vi "Simple example.vi"() -> ()   [LabVIEW 2020]
uses:
  shared/OnOffTypeDef.ctl
  Serial Commands Slink.ctl
  Gentec SlinkUSB.lvclass
panel:
  out "Measure":dbl format="%.3e"
  out "String":string
  in  "stop new":bool
  out "Ch 2 out":dbl format="%.6f"
  in  "error in (no error)":errorcluster
  out "Channel 1 value":dbl
  out "Channel 2 value":dbl
  out "Message Based Settings:Termination Character":u8=10 format="%x"
  out "read buffer 5":string
  out "read buffer 4":string
  out "read buffer 3":string
  out "read buffer 2":string
  out "return count 3":u32
  out "return count 2":u32
  out "Scale Ch":dbl format="%^.0e"
  out "Ext Trig":string
  out "Wavelength":string="0"
  out "error out":errorcluster={"status"=TRUE, "code"=-1073807339, "source"="VISA Read in slink read energy w termination chars.vi->Simple example.vi"}
  out "read buffer":string
  in  "stop":bool
  in  "time to reset":i32=1000
  in  "ChannelEnable":cluster{"Channel 1":T1, "Channel 2":T1}={"Channel 1"=enum."on", "Channel 2"=enum."on"}
  in  "devport":string="COM5"
  out "VISA Refnum out":refnum<visa-resource-name>="COM5"
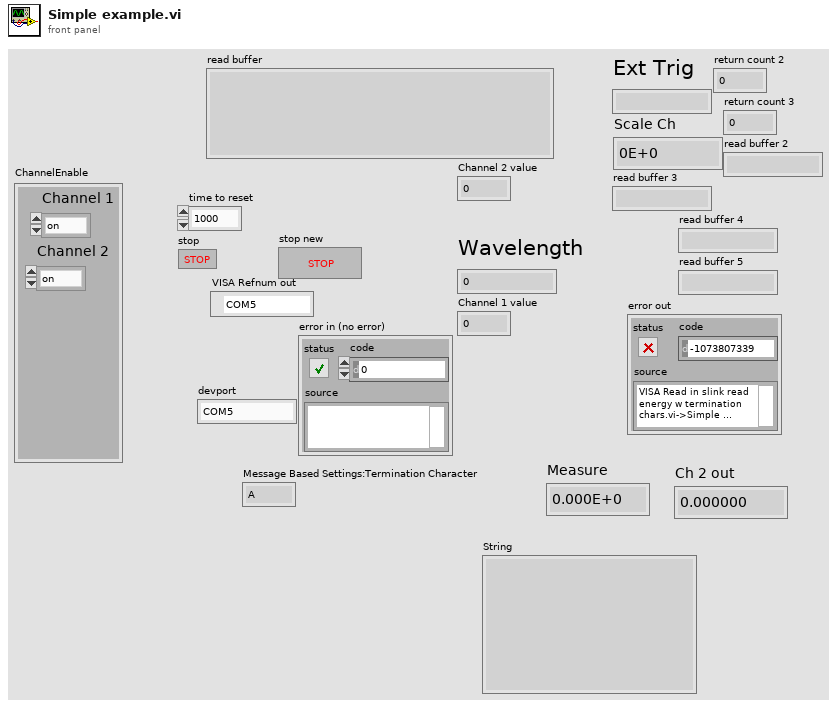
[diagram p1: front panel]
types:
  T1 = typedef "OnOffTypeDef.ctl" = enum16{"off", "on"}
  T2 = typedef "Serial Commands Slink.ctl" = i32
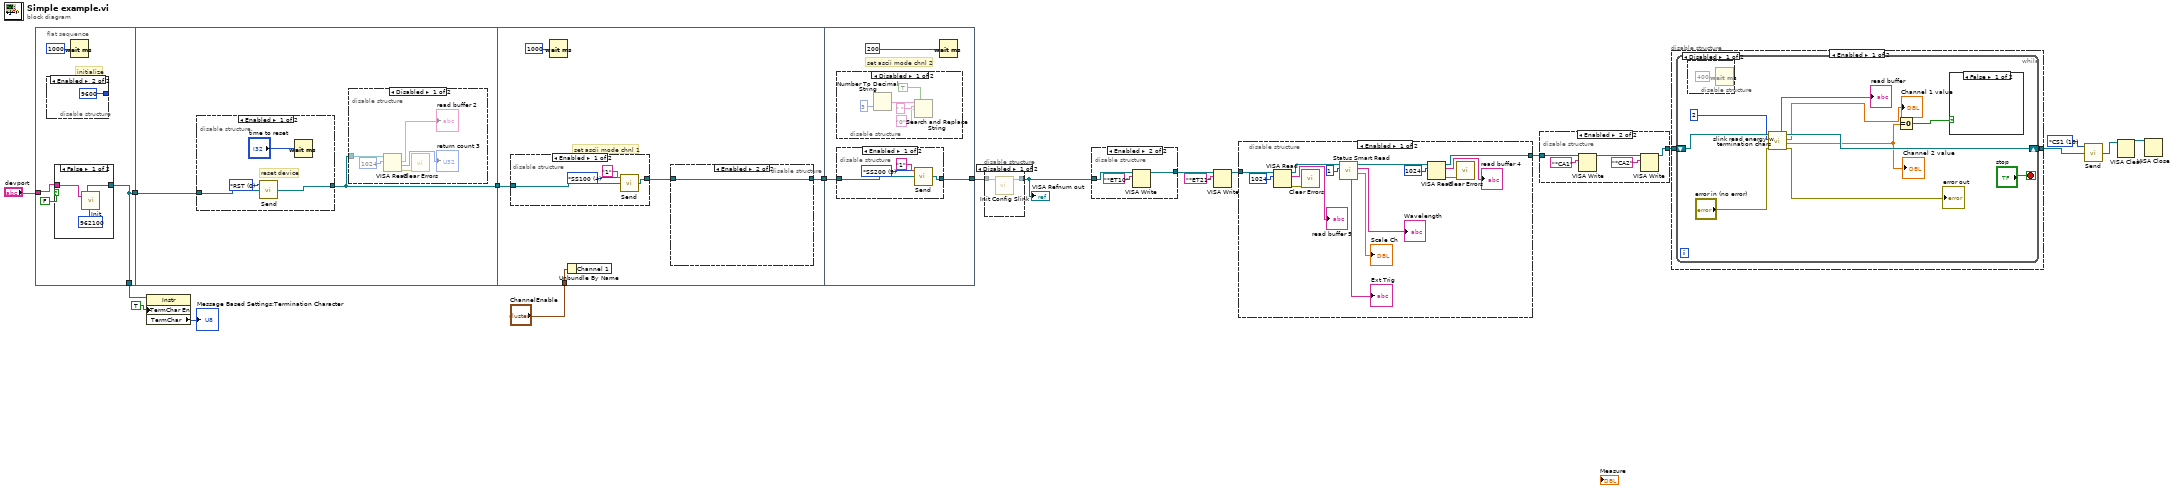
[diagram p0: block diagram]
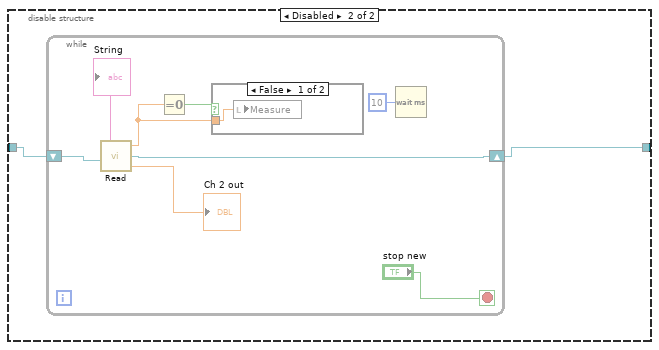
[diagram p4: hidden frame]
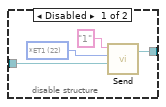
[diagram p7: hidden frame]
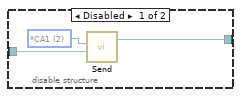
[diagram p9: hidden frame]
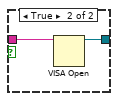
[diagram p10: hidden frame]
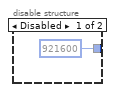
[diagram p11: hidden frame]
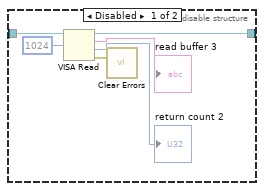
[diagram p14: hidden frame]
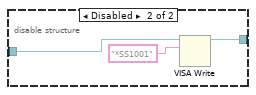
[diagram p15: hidden frame]
diagram:
  w11 = 10 items=["*RST", "*VER", "*CA1", "*CA2", "*SS1", "*SS2", "*SU1", "*SU2", "*SD1", "*SD2", "*CS1", "*CS2", "*AT1", "*AT2", "*AN1", "*AN2", "*PW1", "*PW2", "*TL1", "*TL2", "*ST1", "*ST2", "*ET1", "*ET2", "*EM1", "*EM2", "*SC1", "*SC2"] ("string to write")
  n1 = flat-sequence {
    tunnel: "devport" -> [w22]
    tunnel: [w21] -> w19
    tunnel: [w21] -> w6
    tunnel: w19 -> [w32]
    tunnel: [w31] -> w18
    tunnel: w18 -> [w46]
    tunnel: [w43] -> w17
    tunnel: "ChannelEnable" -> [w45]
    tunnel: [w63] -> w14
    tunnel: w17 -> [w62]
    frame #0 {
      # "initialize"
      n2 = disable-structure shown="Enabled" {
        disable-tunnel: [u32 921600 ("Baud Rate 3") u32 9600 ("Baud Rate 2")] -> _
        frame Disabled {
        }
        frame Enabled {
        }
      }
      n3 = case shown="False" FALSE {
        tunnel: w22 -> [w26 w28]
        tunnel: [w25 w27] -> w21
        frame False {
          n4 = call "Init.vi"("Baud Rate 2"=u32 962100, "# Port"=w26) -> ("VISA resource name out"=w25:refnum<visa-resource-name>)
        }
        frame True {
          n5 = VISA Open(VISA resource name=w28) -> (VISA resource name=w27:refnum<visa-resource-name>)  [unwired: 4 in, 1 out]
        }
      }
      n6 = Wait (ms)(milliseconds to wait=1000) -> ()  [unwired: 1 out]
    }
    frame #1 {
      n7 = disable-structure shown="Enabled" {
        disable-tunnel: [w40 w42] -> w31
        disable-tunnel: w32 -> [w39 w42]
        frame Enabled {
          w38 = T2 0 items=["*RST", "*VER", "*CA1", "*CA2", "*SS100", "*SS200", "*SU1", "*SU2", "*SD1", "*SD2", "*CS1", "*CS2", "*AT1", "*AT2", "*AN1", "*AN2", "*PW1", "*PW2", "*TL1", "*TL2", "*ST1", "*ST2", "*ET1", "*ET2", "*EM1", "*EM2", "*SC1", "*SC2", "*VNM", "*CV1", "*CV2"] ("string to write")
          # "reset device"
          n8 = call "Send.vi"("string to write"=w38, "port number"=w39) -> ("VISA resource name out"=w40:refnum<visa-resource-name>)  [unwired: 2 in, 1 out]
          n9 = Wait (ms)(milliseconds to wait="time to reset") -> ()  [unwired: 1 out]
        }
        frame Disabled {
        }
      }
      n10 = disable-structure shown="Disabled" {
        disable-tunnel: w31 -> [w36 _]
        frame Disabled {
          n11 = VISA Read(VISA resource name=w36, byte count=u32 1024) -> (read buffer=→"read buffer 2":string, return count=→"return count 3":u32, error out=w35:errorcluster)  [unwired: 1 in, 1 out]
          n12 = call <vilib>:"Clear Errors.vi"("error in (no error)"=w35) -> ()  [unwired: 5 in, 2 out]
        }
        frame Enabled {
        }
      }
    }
    frame #2 {
      # "set ascii mode chnl 1"
      n13 = disable-structure shown="Enabled" {
        disable-tunnel: w46 -> [w58 w60]
        disable-tunnel: [w56 w59] -> w44
        frame Enabled {
          w55 = T2 4 items=["*RST", "*VER", "*CA1", "*CA2", "*SS100", "*SS200", "*SU1", "*SU2", "*SD1", "*SD2", "*CS1", "*CS2", "*AT1", "*AT2", "*AN1", "*AN2", "*PW1", "*PW2", "*TL1", "*TL2", "*ST1", "*ST2", "*ET1", "*ET2", "*EM1", "*EM2", "*SC1", "*SC2", "*VNM", "*CV1", "*CV2"] ("string to write")
          n14 = call "Send.vi"("string to write"=w55, "port number"=w58, "Option"="1") -> ("VISA resource name out"=w56:refnum<visa-resource-name>)  [unwired: 1 in, 1 out]
        }
        frame Disabled {
          n15 = VISA Write(VISA resource name=w60, write buffer="*SS1001") -> (VISA resource name out=w59:refnum<visa-resource-name>)  [unwired: 1 in, 2 out]
        }
      }
      n16 = Wait (ms)(milliseconds to wait=1000) -> ()  [unwired: 1 out]
      n17 = Unbundle By Name(w45) -> ()  [unwired: 1 out]
      n18 = disable-structure shown="Enabled" {
        disable-tunnel: w44 -> [w51 w54]
        disable-tunnel: [w48 w54] -> w43
        frame Disabled {
          n19 = VISA Read(VISA resource name=w51, byte count=u32 1024) -> (VISA resource name out=w48:refnum<visa-resource-name>, read buffer=→"read buffer 3":string, return count=→"return count 2":u32, error out=w52:errorcluster)  [unwired: 1 in]
          n20 = call <vilib>:"Clear Errors.vi"("error in (no error)"=w52) -> ()  [unwired: 5 in, 2 out]
        }
        frame Enabled {
        }
      }
    }
    frame #3 {
      # "set ascii mode chnl 2"
      n21 = disable-structure shown="Disabled" {
        frame Disabled {
          n22 = Number To Decimal String(width (-)=i16 3) -> (decimal integer string=w73:string)  [unwired: 1 in]
          n23 = Search and Replace String(replace all?=TRUE ("replace all? (F)"), input string=w73, search string=" ", replace string="0" ("replace string (\"\")")) -> ()  [unwired: 4 in, 4 out]
        }
        frame Enabled {
        }
      }
      n24 = disable-structure shown="Enabled" {
        disable-tunnel: [w68 w69] -> w63
        disable-tunnel: w62 -> [w67 w69]
        frame Enabled {
          w65 = T2 5 items=["*RST", "*VER", "*CA1", "*CA2", "*SS100", "*SS200", "*SU1", "*SU2", "*SD1", "*SD2", "*CS1", "*CS2", "*AT1", "*AT2", "*AN1", "*AN2", "*PW1", "*PW2", "*TL1", "*TL2", "*ST1", "*ST2", "*ET1", "*ET2", "*EM1", "*EM2", "*SC1", "*SC2", "*VNM", "*CV1", "*CV2"] ("string to write")
          n25 = call "Send.vi"("string to write"=w65, "port number"=w67, "Option"="1" ("search string")) -> ("VISA resource name out"=w68:refnum<visa-resource-name>)  [unwired: 1 in, 1 out]
        }
        frame Disabled {
        }
      }
      n26 = Wait (ms)(milliseconds to wait=200) -> ()  [unwired: 1 out]
    }
  }
  n27 = property class="Instr"(reference=w6, "TermChar En"=TRUE ("Message Based Settings:Termination Character Enable")) -> ("TermChar"=→"Message Based Settings:Termination Character":u8)  [unwired: 1 in, 2 out]
  n28 = disable-structure shown="Disabled" {
    disable-tunnel: w14 -> [w76 w77]
    disable-tunnel: [w75 w77] -> w12
    frame Disabled {
      n29 = call "Init Config Slink.vi"("VISA Refnum in"=w76) -> ("VISA Refnum out"=w75:refnum<visa-resource-name>)  [unwired: 9 in, 1 out]
    }
    frame Enabled {
    }
  }
  "VISA Refnum out" <- w12
  n30 = disable-structure shown="Enabled" {
    disable-tunnel: w12 -> [w80 w83]
    disable-tunnel: [w78 w82] -> w2
    frame Disabled {
      w81 = 22 items=["*RST", "*VER", "*CA1", "*CA2", "*SS1", "*SS2", "*SU1", "*SU2", "*SD1", "*SD2", "*CS1", "*CS2", "*AT1", "*AT2", "*AN1", "*AN2", "*PW1", "*PW2", "*TL1", "*TL2", "*ST1", "*ST2", "*ET1", "*ET2", "*EM1", "*EM2", "*SC1", "*SC2"] ("string to write")
      n31 = call "Send.vi"("port number"=w80, "string to write"=w81, "Option"="1") -> ("port out"=w78:refnum<visa-resource-name>)  [unwired: 1 in, 1 out]
    }
    frame Enabled {
      n32 = VISA Write(VISA resource name=w83, write buffer="*ET10") -> (VISA resource name out=w82:refnum<visa-resource-name>)  [unwired: 1 in, 2 out]
    }
  }
  n33 = VISA Write(VISA resource name=w2, write buffer="*ET21") -> (VISA resource name out=w1:refnum<visa-resource-name>)  [unwired: 1 in, 2 out]
  n34 = disable-structure shown="Enabled" {
    disable-tunnel: w1 -> [w92 w99]
    disable-tunnel: [w87 w99] -> w7
    frame Enabled {
      n35 = VISA Read(VISA resource name=w92, byte count=u32 1024) -> (VISA resource name out=w91:refnum<visa-resource-name>, read buffer=→"read buffer 5":string, error out=w93:errorcluster)  [unwired: 1 in, 1 out]
      n36 = call <vilib>:"Clear Errors.vi"("error in (no error)"=w93) -> ()  [unwired: 5 in, 2 out]
      n37 = call "Status Smart Read.vi"("Channel"=1, "Com Port"=w91) -> ("Scale Ch"=→"Scale Ch":dbl, "wavelengt dec string"=→"Wavelength":string, "VISA Refnum out"=w88:refnum<visa-resource-name>, "Ext Trig"=→"Ext Trig":string)  [unwired: 4 in, 2 out]
      n38 = VISA Read(VISA resource name=w88, byte count=u32 1024) -> (VISA resource name out=w87:refnum<visa-resource-name>, read buffer=→"read buffer 4":string, error out=w89:errorcluster)  [unwired: 1 in, 1 out]
      n39 = call <vilib>:"Clear Errors.vi"("error in (no error)"=w89) -> ()  [unwired: 5 in, 2 out]
    }
    frame Disabled {
    }
  }
  n40 = disable-structure shown="Enabled" {
    disable-tunnel: w7 -> [w101 w106]
    disable-tunnel: [w100 w103] -> w13
    frame Disabled {
      w102 = 2 items=["*RST", "*VER", "*CA1", "*CA2", "*SS1", "*SS2", "*SU1", "*SU2", "*SD1", "*SD2", "*CS1", "*CS2", "*AT1", "*AT2", "*AN1", "*AN2", "*PW1", "*PW2", "*TL1", "*TL2", "*ST1", "*ST2", "*ET1", "*ET2", "*EM1", "*EM2", "*SC1", "*SC2"] ("string to write")
      n41 = call "Send.vi"("port number"=w101, "string to write"=w102) -> ("port out"=w100:refnum<visa-resource-name>)  [unwired: 2 in, 1 out]
    }
    frame Enabled {
      n42 = VISA Write(VISA resource name=w106, write buffer="*CA1") -> (VISA resource name out=w104:refnum<visa-resource-name>)  [unwired: 1 in, 2 out]
      n43 = VISA Write(VISA resource name=w104, write buffer="*CA2") -> (VISA resource name out=w103:refnum<visa-resource-name>)  [unwired: 1 in, 2 out]
    }
  }
  n44 = disable-structure shown="Enabled" {
    disable-tunnel: w13 -> [w109 w122]
    disable-tunnel: [w108 w121] -> w10
    frame Enabled {
      n45 = while {
        shift-right: [w114] -> w108
        shift-left: w109 -> [w118]
        stop <- "stop" stop-if-true
        n46 = disable-structure shown="Disabled" {
          frame Disabled {
            n47 = Wait (ms)(milliseconds to wait=u32 400) -> ()  [unwired: 1 out]
          }
          frame Enabled {
          }
        }
        n48 = call "slink read energy w termination chars.vi"("error in (no error)"="error in (no error)", "# channels"=2, "VISA Refnum in"=w118) -> ("error out"=→"error out":errorcluster, "Channel 2 value"=w110:dbl, "Channel 1 value"=→"Channel 1 value":dbl, "VISA Refnum out"=w114:refnum<visa-resource-name>, "String"=→"read buffer":string)  [unwired: 4 in]
        "Channel 2 value" <- w110
        n49 = Equal To 0?(x=w110) -> (x = 0?=w116:bool)
        n50 = case shown="False" w116 {
          frame False {
          }
          frame True {
          }
        }
      }
    }
    frame Disabled {
      n51 = while {
        shift-right: [w127] -> w121
        shift-left: w122 -> [w128]
        stop <- "stop new" stop-if-true
        n52 = call "Read.vi"("Com Port"=w128) -> ("Ch 2 out"=→"Ch 2 out":dbl, "Com out"=w127:refnum<visa-resource-name>, "Ch 1 out"=w123:dbl, "String"=→"String":string)  [unwired: 2 in]
        n53 = Equal To 0?(x=w123) -> (x = 0?=w124:bool)
        n54 = case shown="False" w124 {
          tunnel: w123 -> [w131 _]
          frame False {
            n55 = local write "Measure"(w131) -> ()
          }
          frame True {
          }
        }
        n56 = Wait (ms)(milliseconds to wait=u32 10) -> ()  [unwired: 1 out]
      }
    }
  }
  n57 = call "Send.vi"("string to write"=w11, "port number"=w10) -> ("VISA resource name out"=w9:refnum<visa-resource-name>)  [unwired: 2 in, 1 out]
  n58 = VISA Clear(VISA resource name=w9) -> (VISA resource name out=w8:refnum<visa-resource-name>)  [unwired: 1 in, 1 out]
  n59 = VISA Close(VISA resource name=w8) -> ()  [unwired: 1 in, 1 out]
